vi "p5.3.vi"() -> ()   [LabVIEW 2020]
uses:
  <vilib>/Analysis/NI_AALBase.lvlib
panel:
  out "A (db)":dbl=20.0
  out "N+1":i32=9
  out "Y":dbl[](graph)
  out "DFT Y":dbl[](graph)
  out "DFT X":dbl[](graph)
  out "X":dbl[](graph)
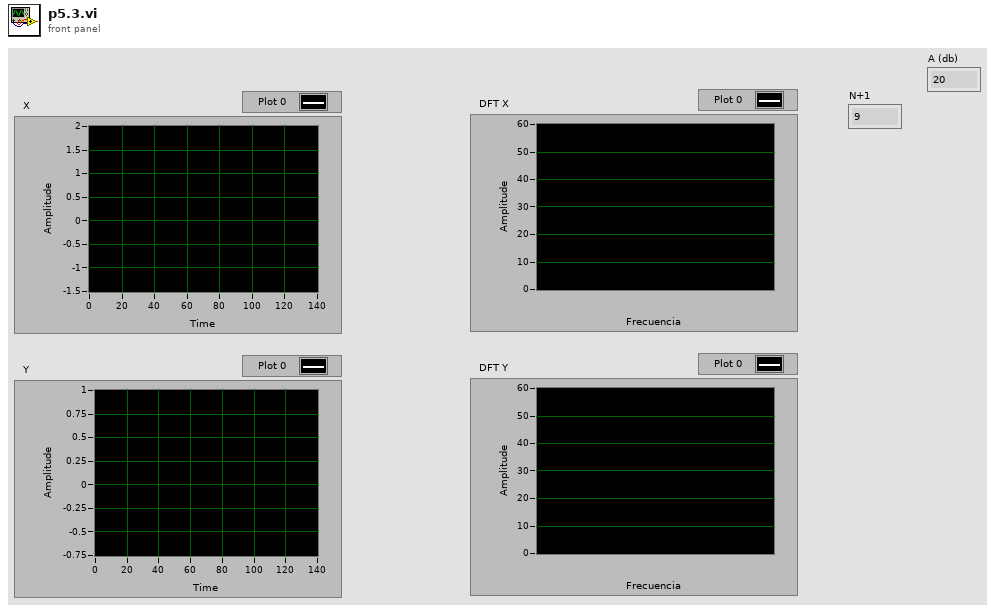
[diagram p1: front panel]
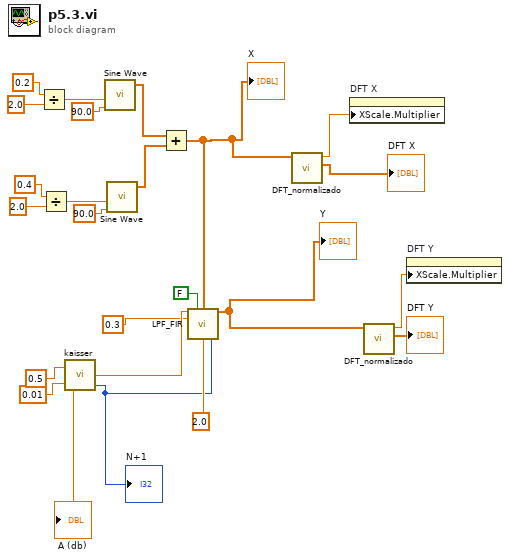
[diagram p0: block diagram]
diagram:
  n1 = Divide(x=0.2, y=2.0) -> (x/y=w19:dbl)
  n2 = Divide(x=0.4, y=2.0) -> (x/y=w18:dbl)
  n3 = call "kaisser.vi"("Banda Transicion (normalizada)"=0.5, "delta (rizado)"=0.01) -> ("A (db)"=→"A (db)":dbl, "Beta"=w7:dbl, "N+1"=w2:i32)
  "N+1" <- w2
  n4 = call <vilib>:"Sine Wave.vi"("frequency"=w19, "phase in"=90.0) -> ("sine wave"=w14:dbl[])  [unwired: 3 in, 2 out]
  n5 = call <vilib>:"Sine Wave.vi"("frequency"=w18, "phase in"=90.0) -> ("sine wave"=w13:dbl[])  [unwired: 3 in, 2 out]
  n6 = Add(x=w14, y=w13) -> (x+y=w11:dbl[])
  "X" <- w11
  n7 = call "LPF_FIR.vi"("window parameter"=w7, "init/cont (init:F)"=FALSE, "Array"=w11, "low cutoff freq: fl"=0.3 ("high cutoff freq: fh"), "sampling freq: fs"=2.0, "taps"=w2) -> ("Filtered X"=w8:dbl[])  [unwired: 9 in]
  "Y" <- w8
  n8 = call "DFT_normalizado.vi"("X"=w11) -> ("Array"=→"DFT X":dbl[], "Numeric"=w22:dbl)  [unwired: 9 in]
  n9 = property on="DFT X" class="WFGraph (strict)"("XScale.Multiplier"=w22) -> ()  [unwired: 2 in, 2 out]
  n10 = call "DFT_normalizado.vi"("X"=w8) -> ("Array"=→"DFT Y":dbl[], "Numeric"=w10:dbl)  [unwired: 9 in]
  n11 = property on="DFT Y" class="WFGraph (strict)"("XScale.Multiplier"=w10) -> ()  [unwired: 2 in, 2 out]
